vi "Lab1.vi"() -> ()   [LabVIEW 2011]
panel:
  out "Indicator":dbl
  in  "Control2":dbl
  in  "Control1":dbl
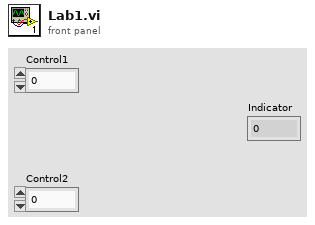
[diagram p1: front panel]
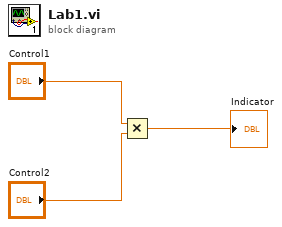
[diagram p0: block diagram]
diagram:
  n1 = Multiply(x="Control1", y="Control2") -> (x*y=→"Indicator":dbl)
